vi "Bead threshold manual adjust 2.vi"(6 "Standalone(F)":bool, 7 "error in (no error)":errorcluster, 10 "Image In":T3) -> (0 "error out":errorcluster, 1 "enclosure box":T1 {"Rotation" format="%.2f"; "Left" scale=0.0..1024.0; "Right" scale=0.0..1024.0}, 2 "Centroid array":T4(array[cluster]), 3 "Source Image":T3(plugin-control) caption="Threshold Image")   [LabVIEW 2020]
uses:
  <vilib>/vision/Image Controls.llb/IMAQ Image.ctl
  <vilib>/vision/NI_Vision_Development_Module.lvlib
panel:
  out "Histogram":T2(graph)
  out "error out 2":errorcluster
  in  "Boundary":i16
  out "Centroid":cluster{"X Centroid":sgl, "Y Centroid":sgl} {"Y Centroid" format="%.2f"; "X Centroid" format="%.2f"}
  out "Reference Rectangles":i16[][](array[numeric])
  out "Number of Particles":i32
  in  "Morphology Iterations":i32=1
  in  "Morphology Operation":T5(ring)=enum."Erode"
  in  "Adjust Separation":i32=3 min=3
  in  "Threshold":cluster{sgl, sgl}(slide)={0.0, 168.81285} scale=0.0..255.0
  out "Color Palette out":cluster{"Red":u8, "Green":u8, "Blue":u8}[](array[cluster])
  in  "File Path":path
  in  "stop":bool
  out "Image Show Binary":T3(plugin-control)
  out "Selected Rectangle":i16[](array[numeric])
  out "Image Pixels (I16)":i16[][](array[numeric])
  out "Image Pixels (U8)":u8[][](array[numeric])
  out "Image Pixels (Float)":sgl[][](array[numeric]) format="%.2f"
  out "Image Pixels (U16)":u16[][](array[numeric])
  out "Source Image":T3(plugin-control) caption="Threshold Image"
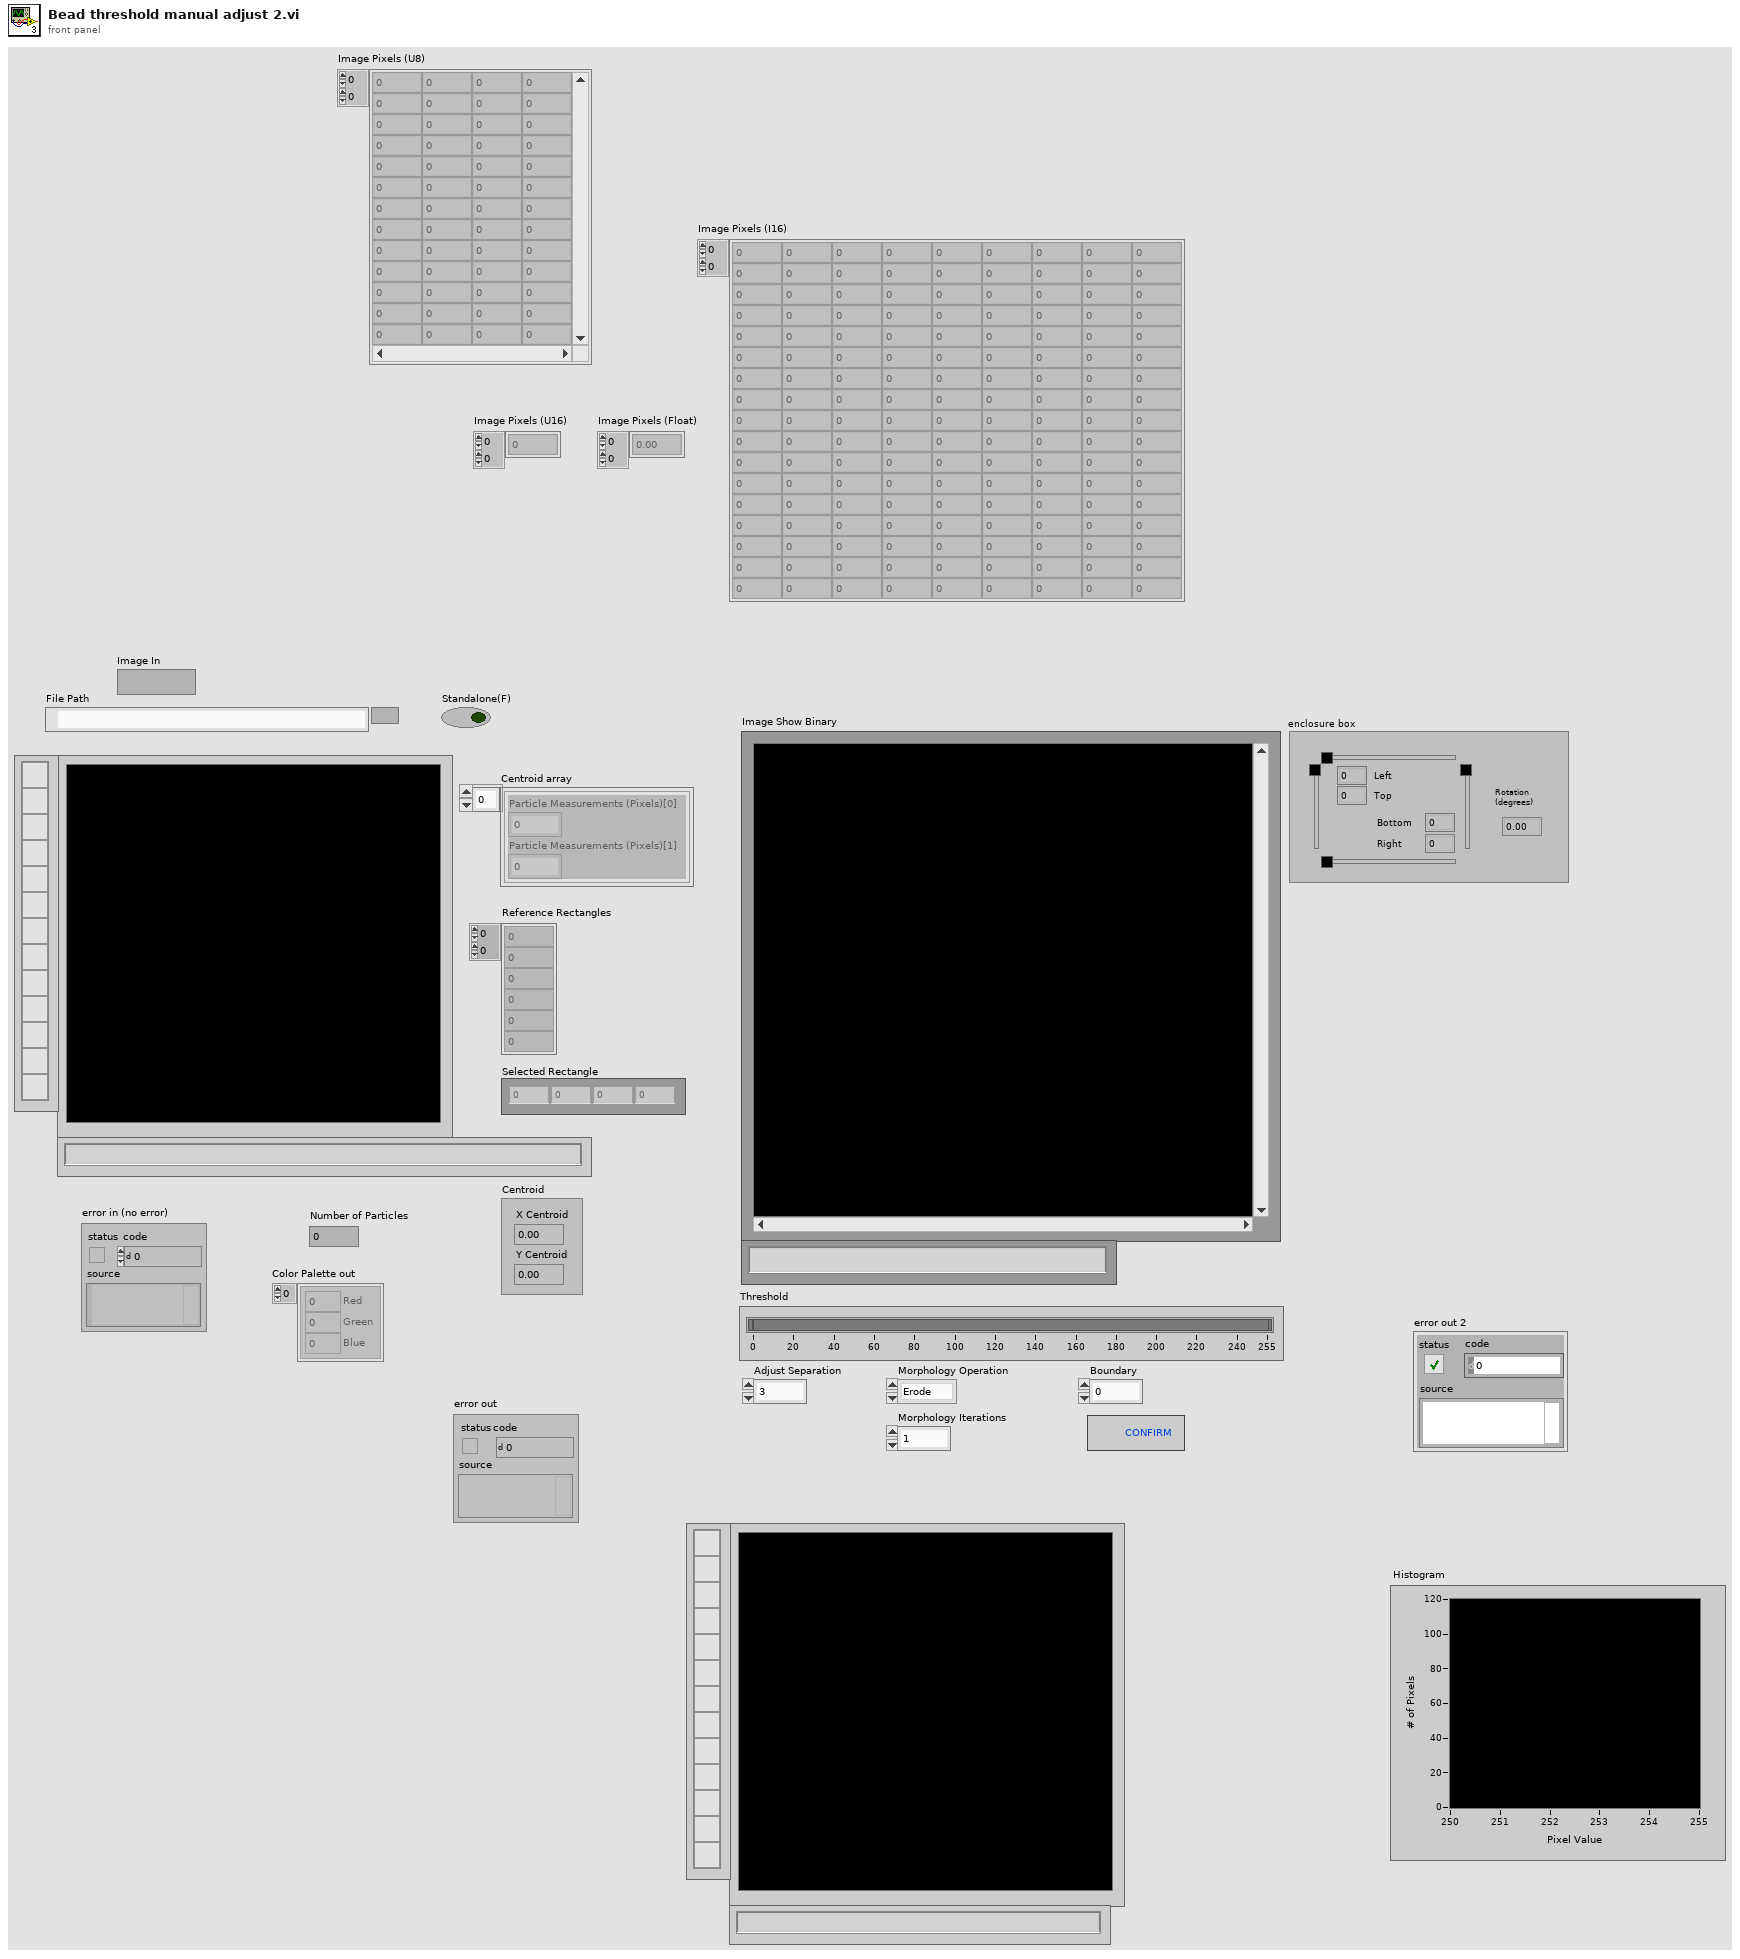
[diagram p1: front panel]
types:
  T1 = typedef "IMAQ Rectangle" = cluster{"Left":i32, "Top":i32, "Right":i32, "Bottom":i32, "Rotation":dbl}
  T2 = cluster{"Starting Value":sgl, "Incremental Value":sgl, "Histogram":u32[]}
  T3 = typedef "IMAQ Image.ctl" = refnum<image>
  T4 = cluster{"Particle Measurements (Pixels)[0]":dbl, "Particle Measurements (Pixels)[1]":dbl}[]
  T5 = enum32{"AutoM", "Close", "Dilate", "Erode", "Gradient", "Gradient out", "Gradient in", "Hit miss", "Open", "PClose", "POpen", "Thick", "Thin"}
  T6 = typedef "Image Type" = u32
  T7 = cluster{"Global Rectangle":i32[], "Contours":cluster{"Contour Type":u32, "ROI Type":u32, "Points":i32[]}[]}
  T8 = cluster{"Left":i32, "Top":i32, "Right":i32, "Bottom":i32}
  T9 = cluster{"Particle Measurements (Pixels)[0]":dbl, "Particle Measurements (Pixels)[1]":dbl}
  T10 = typedef "Particle Parameters" = i32
  T11 = typedef "ROI Descriptor" = cluster{"Global Rectangle":i32[], "Contours":cluster{"ID":enum32{"External", "Internal"}, "Type":u32, "Coordinates":i32[]}[]}
  T12 = cluster{"Measurement Parameter":T10, "Range Lower Value":dbl, "Range Upper Value":dbl, "Range":bool, "Measurement Type":bool}
  T13 = cluster{"Measurement Parameter":T10, "Range Lower Value":dbl, "Range Upper Value":dbl, "Range":bool, "Measurement Type":bool}[]
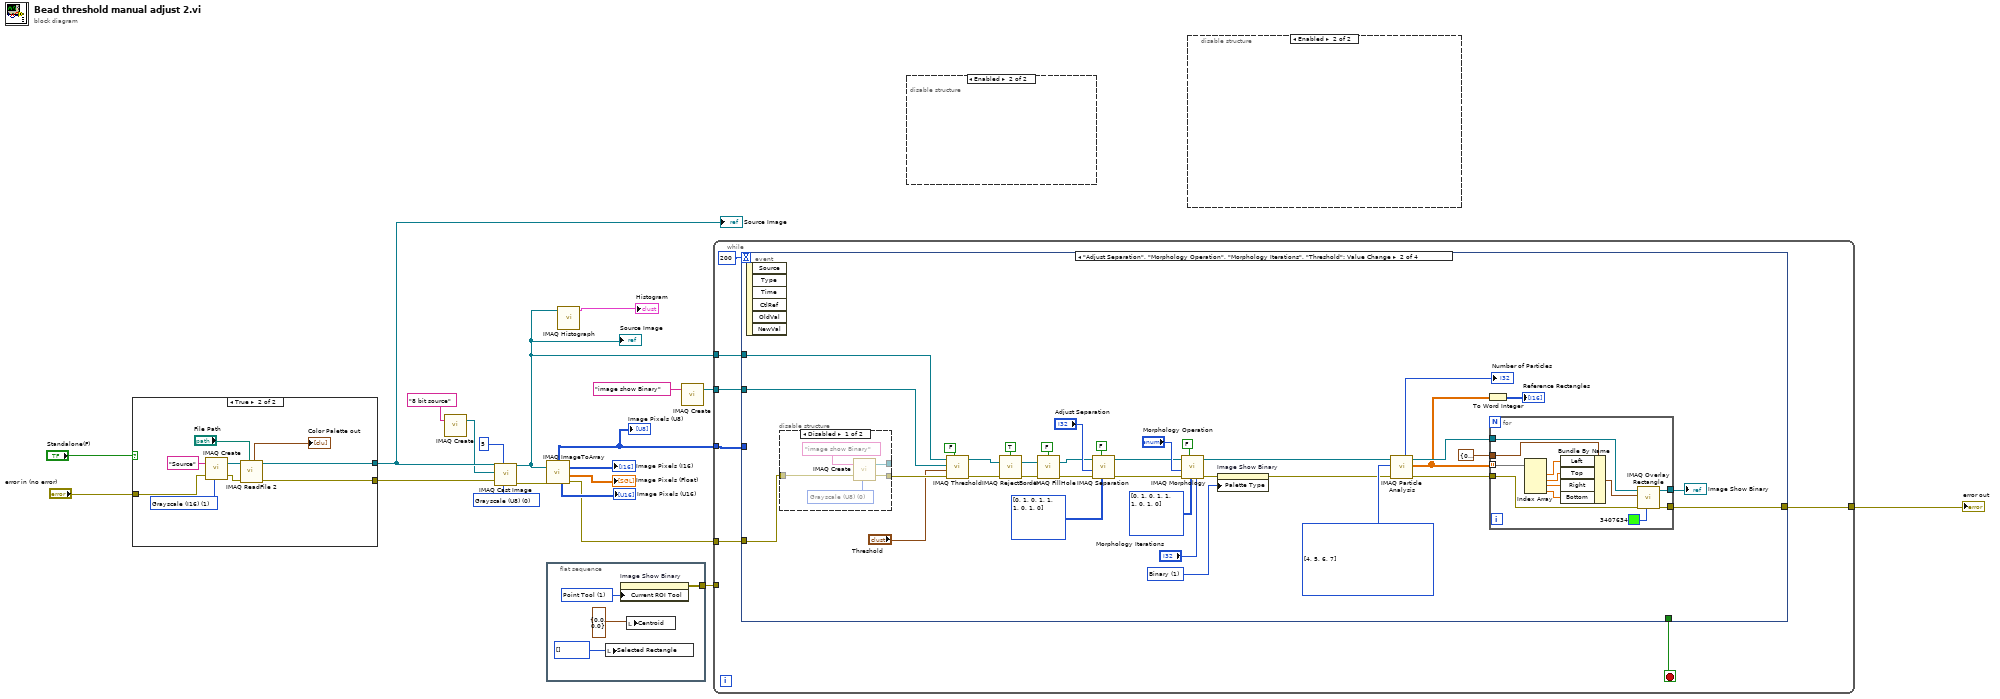
[diagram p0: block diagram]
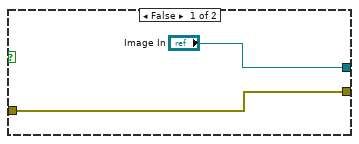
[diagram p2: hidden frame]
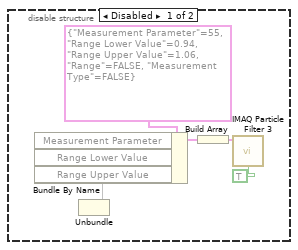
[diagram p3: hidden frame]
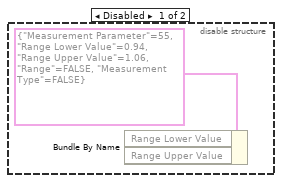
[diagram p4: hidden frame]
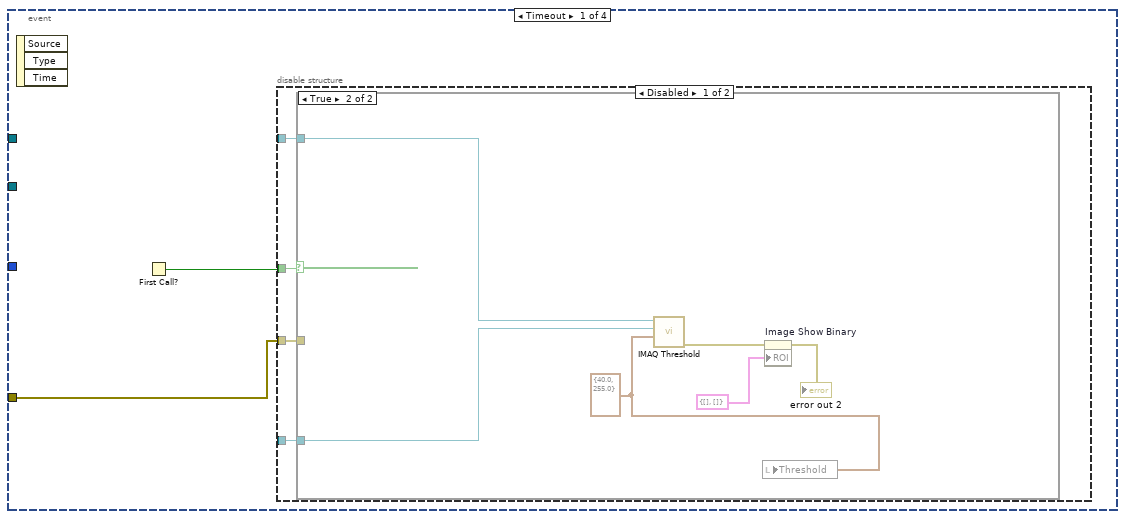
[diagram p5: hidden frame]
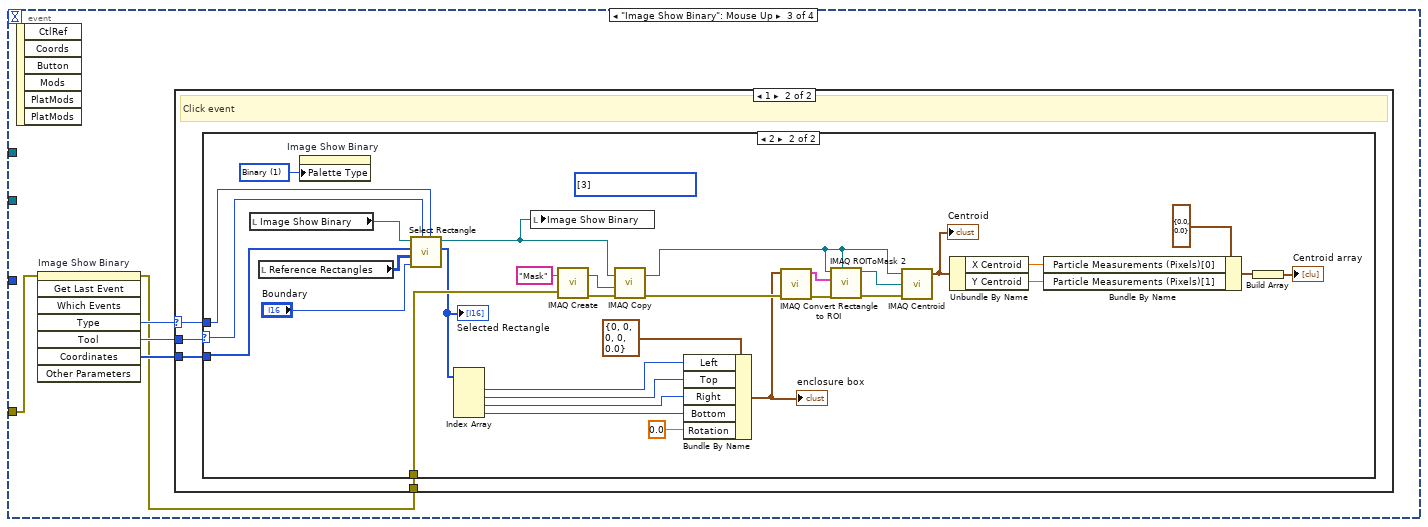
[diagram p9: hidden frame]
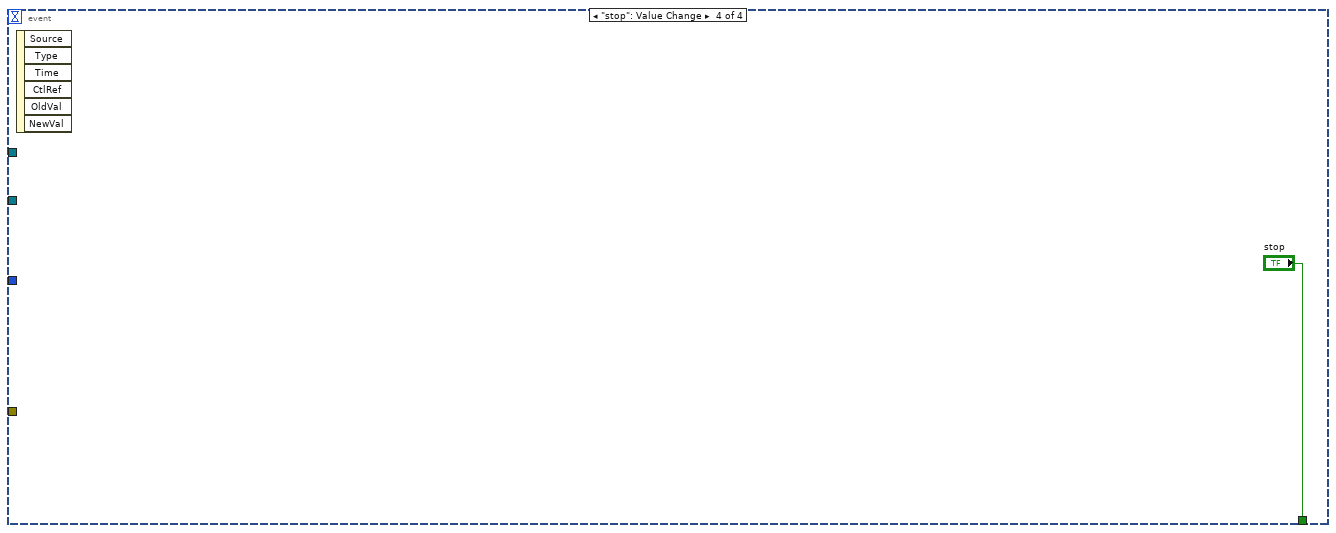
[diagram p12: hidden frame]
diagram:
  w7 = T6 0 items=["Grayscale (U8)", "Grayscale (I16)", "Grayscale (SGL)", "Complex (CSG)", "RGB (U32)", "HSL (U32)", "RGB (U64)", "Grayscale (U16)"] ("Image Type")
  n1 = case shown="True" "Standalone(F)" {
    tunnel: ["Image In" w24] -> w8
    tunnel: "error in (no error)" -> [w22 w25]
    tunnel: [w22 w23] -> w10
    frame False {
    }
    frame True {
      w31 = T6 1 items=["Grayscale (U8)", "Grayscale (I16)", "Grayscale (SGL)", "Complex (CSG)", "RGB (U32)", "HSL (U32)", "RGB (U64)", "Grayscale (U16)"] ("Image Type")
      n2 = call "IMAQ Create"("Image Name"="Source", "Image Type"=w31, "error in (no error)"=w25) -> ("New Image"=w29:T3, "error out"=w26:errorcluster)  [unwired: 2 in]
      n3 = call "IMAQ ReadFile 2"("File Path"="File Path", "error in (no error)"=w26, "Image"=w29) -> ("error out"=w23:errorcluster, "Image Out"=w24:T3, "Color Palette out"=→"Color Palette out":cluster{"Red":u8, "Green":u8, "Blue":u8}[])  [unwired: 4 in, 2 out]
    }
  }
  "Source Image" <- w8
  n4 = call "IMAQ Create"("Image Name"="8 bit source") -> ("New Image"=w2:T3)  [unwired: 4 in, 1 out]
  n5 = call "IMAQ Cast Image"("Image Type"=w7, "# Shifts"=5, "error in (no error)"=w10, "Image Dst"=w2, "Image Src"=w8) -> ("error out"=w9:errorcluster, "Image Dst Out"=w1:T3)  [unwired: 5 in]
  "Source Image" <- w1
  n6 = flat-sequence {
    tunnel: [w34] -> w12
    frame #0 {
      w35 = u32 1 items=["Zoom Tool"=8, "Selection Tool"=0, "Pan Tool"=9, "Point Tool"=1, "Line Tool"=2, "Rectangle Tool"=3, "Rotated Rectangle Tool"=12, "Polyline Tool"=10, "Polygon Tool"=5, "Freehand Tool"=11, "Closed Freehand Tool"=6, "Ellipse Tool"=4, "Annulus Tool"=7] ("Current ROI Tool")
      n7 = local write "Selected Rectangle"(i16[] []) -> ()
      n8 = property on="Image Show Binary" class="ImageControl"("Current ROI Tool"=w35) -> (error out=w34:errorcluster)  [unwired: 2 in, 1 out]
      n9 = local write "Centroid"(cluster{"X Centroid":sgl, "Y Centroid":sgl} {"X Centroid"=0.0, "Y Centroid"=0.0} ("Centroid")) -> ()
    }
  }
  n10 = call "IMAQ ImageToArray"("error in (no error)"=w9, "Image"=w1) -> ("Image Pixels (U16)"=→"Image Pixels (U16)":u16[][], "Image Pixels (Float)"=→"Image Pixels (Float)":sgl[][], "error out"=w15:errorcluster, "Image Pixels (U8)"=w17:u8[][], "Image Pixels (I16)"=→"Image Pixels (I16)":i16[][])  [unwired: 2 in]
  "Image Pixels (U8)" <- w17
  n11 = call "IMAQ Histograph"("Image"=w1) -> ("Histogram Graph"=→"Histogram":T2)  [unwired: 7 in, 3 out]
  n12 = call "IMAQ Create"("Image Name"="image show Binary") -> ("New Image"=w4:T3)  [unwired: 4 in, 1 out]
  n13 = while {
    tunnel: w17 -> [w42]
    tunnel: w1 -> [w39]
    tunnel: [w38] -> w16
    tunnel: w15 -> [w37]
    tunnel: w12 -> [_]
    tunnel: w4 -> [w36]
    stop <- w41 stop-if-true
    n14 = event shown="[1] \"Adjust Separation\", \"Morphology Operation\", \"Morphology Iterations\", \"Threshold\": Value Change" {
      selector: _ -> [_ _ _ _]
      dyn-events: _ -> [_ _ _ _]
      timeout: 200 -> [_ _ _ _]
      tunnel: w42 -> [_ _ _ _]
      tunnel: [_ _ _ "stop"] -> w41
      tunnel: w39 -> [_ w58 _ _]
      tunnel: [_ w63 _ _] -> w38
      tunnel: w37 -> [w43 w62 w110 _]
      tunnel: w36 -> [_ w57 _ _]
      event Timeout {
        n15 = event-data() -> ()  [unwired: 1 in, 3 out]
        n16 = First Call?() -> (First Call?: T/F=w44:bool)
        n17 = disable-structure shown="Disabled" {
          disable-tunnel: w44 -> [w48 _]
          disable-tunnel: _ -> [w47 _]
          disable-tunnel: w43 -> [w46 _]
          disable-tunnel: _ -> [w45 _]
          frame Disabled {
            n18 = case shown="True" w48 {
              tunnel: w47 -> [_ w50]
              tunnel: w46 -> [_ _]
              tunnel: w45 -> [_ w49]
              frame False {
              }
              frame True {
                w51 = cluster{"Lower value":sgl, "Upper value":sgl} {"Lower value"=40.0, "Upper value"=255.0} ("Range")
                n19 = call "IMAQ Threshold"("Range"=w51, "Image Dst"=w49, "Image Src"=w50) -> ("error out"=w53:errorcluster)  [unwired: 7 in, 1 out]
                n20 = local write "Threshold"(w51) -> ()
                n21 = property on="Image Show Binary" class="ImageControl"(error in=w53, "ROI"=T7 {"Global Rectangle"=[], "Contours"=[]}) -> (error out=→"error out 2":errorcluster)  [unwired: 1 in, 1 out]
              }
            }
          }
          frame Enabled {
          }
        }
      }
      event "Adjust Separation", "Morphology Operation", "Morphology Iterations", "Threshold": Value Change {
        w76 = T10[] [4, 5, 6, 7] items=["Center of Mass X", "Center of Mass Y", "First Pixel X", "First Pixel Y", "Bounding Rect Left", "Bounding Rect Top", "Bounding Rect Right", "Bounding Rect Bottom", "Max Feret Diameter Start X", "Max Feret Diameter Start Y", "Max Feret Diameter End X", "Max Feret Diameter End Y", "Max Horiz. Segment Length Left", "Max Horiz. Segment Length Right", "Max Horiz. Segment Length Row", "-", "Bounding Rect Width", "Bounding Rect Height", "Bounding Rect Diagonal", "Perimeter", "Convex Hull Perimeter", "Holes' Perimeter", "Max Feret Diameter", "Equivalent Ellipse Major Axis", "Equivalent Ellipse Minor Axis", "Equivalent Ellipse Minor Axis (Feret)", "Equivalent Rect Long Side", "Equivalent Rect Short Side", "Equivalent Rect Diagonal", "Equivalent Rect Short Side (Feret)", "Average Horiz. Segment Length", "Average Vert. Segment Length", "Hydraulic Radius", "Waddel Disk Diameter", "-", "Area", "Holes' Area", "Particle & Holes' Area", "Convex Hull Area", "Image Area", "-", "Number of Holes", "Number of Horiz. Segments", "Number of Vert. Segments", "-", "Orientation", "Max Feret Diameter Orientation", "-", "% Area/Image Area", "% Area/(Particle & Holes' Area)", "Ratio of Equivalent Ellipse Axes", "Ratio of Equivalent Rect Sides", "-", "Elongation Factor", "Compactness Factor", "Heywood Circularity Factor", "Type Factor", "-", "Sum X", "Sum Y", "Sum XX", "Sum XY", "Sum YY", "Sum XXX", "Sum XXY", "Sum XYY", "Sum YYY", "-", "Moment of Inertia XX", "Moment of Inertia XY", "Moment of Inertia YY", "Moment of Inertia XXX", "Moment of Inertia XXY", "Moment of Inertia XYY", "Moment of Inertia YYY", "Norm. Moment of Inertia XX", "Norm. Moment of Inertia XY", "Norm. Moment of Inertia YY", "Norm. Moment of Inertia XXX", "Norm. Moment of Inertia XXY", "Norm. Moment of Inertia XYY", "Norm. Moment of Inertia YYY", "Hu Moment 1", "Hu Moment 2", "Hu Moment 3", "Hu Moment 4", "Hu Moment 5", "Hu Moment 6", "Hu Moment 7"] ("Pixel Measurements")
        w78 = u32 1 items=["Grayscale", "Binary", "Gradient", "Rainbow", "Temperature", "User Defined", "Binary 16 Bit", "Gradient 16 Bit", "Rainbow 16 Bit", "Temperature 16 Bit", "User Defined 16 Bit"] ("Palette Type")
        n22 = event-data() -> ()  [unwired: 1 in, 6 out]
        n23 = disable-structure shown="Disabled" {
          disable-tunnel: w62 -> [w93 w96]
          disable-tunnel: [w92 _] -> _
          disable-tunnel: [w91 w96] -> w56
          frame Disabled {
            w94 = T6 0 items=["Grayscale (U8)", "Grayscale (I16)", "Grayscale (SGL)", "Complex (CSG)", "RGB (U32)", "HSL (U32)", "RGB (U64)", "Grayscale (U16)"] ("Image Type")
            n24 = call "IMAQ Create"("Image Name"="image show Binary", "Image Type"=w94, "error in (no error)"=w93) -> ("New Image"=w92:T3, "error out"=w91:errorcluster)  [unwired: 2 in]
          }
          frame Enabled {
          }
        }
        n25 = call "IMAQ Threshold"("Keep/Replace Value (Replace)"=FALSE, "error in (no error)"=w56, "Range"="Threshold", "Image Dst"=w57, "Image Src"=w58) -> ("error out"=w79:errorcluster, "Image Dst Out"=w67:T3)  [unwired: 5 in]
        n26 = call "IMAQ RejectBorder"("error in (no error)"=w79, "Image Src"=w67, "Connectivity 4/8 (8)"=TRUE) -> ("error out"=w89:errorcluster, "Image Dst Out"=w66:T3)  [unwired: 1 in, 2 out]
        n27 = call "IMAQ FillHole"("error in (no error)"=w89, "Image Src"=w66, "Connectivity 4/8 (8)"=FALSE) -> ("error out"=w85:errorcluster, "Image Dst Out"=w65:T3)  [unwired: 1 in, 2 out]
        n28 = call "IMAQ Separation"("Structuring Element"=i32[][] [[0, 1, 0], [1, 1, 1], [0, 1, 0]], "Square/Hexa (Square)"=FALSE, "error in (no error)"=w85, "Nb of Erosion"="Adjust Separation", "Image Src"=w65) -> ("error out"=w80:errorcluster, "Image Dst Out"=w64:T3)  [unwired: 1 in, 4 out]
        n29 = call "IMAQ Morphology"("Number of iterations (1)"="Morphology Iterations", "Structuring Element"=i32[][] [[0, 1, 0], [1, 1, 1], [0, 1, 0]], "Square/Hexa (Square)"=FALSE, "error in (no error)"=w80, "Operation"="Morphology Operation", "Image Src"=w64) -> ("error out"=w77:errorcluster, "Image Dst Out"=w68:T3)  [unwired: 1 in, 3 out]
        n30 = property on="Image Show Binary" class="ImageControl"(error in=w77, "Palette Type"=w78) -> (error out=w69:errorcluster)  [unwired: 1 in, 1 out]
        n31 = call "IMAQ Particle Analysis"("error in (no error)"=w69, "Pixel Measurements"=w76, "Image"=w68) -> ("error out"=w72:errorcluster, "Particle Measurements (Pixels)"=w71:dbl[][], "Image Out (duplicate)"=w75:T3, "Number of Particles"=→"Number of Particles":i32)  [unwired: 3 in, 2 out]
        n32 = To Word Integer(number=w71) -> (16bit integer=→"Reference Rectangles":i16[][])
        n33 = for {
          tunnel: [w99] -> w61
          tunnel: w75 -> [w107]
          tunnel: w71 -> [w105] mode=indexing
          tunnel: T8 {"Left"=0, "Top"=0, "Right"=0, "Bottom"=0} ("Rectangle") -> [w106]
          tunnel: [w98] -> w63
          tunnel: w72 -> [w97]
          n34 = Index Array(array=w105) -> (element #1=w103:dbl, element #2=w102:dbl, element #3=w101:dbl, element #4=w100:dbl)  [unwired: 4 in]
          n35 = Bundle By Name(cluster=w106, "Left"=w103, "Top"=w102, "Right"=w101, "Bottom"=w100) -> (w104:T8)
          n36 = call "IMAQ Overlay Rectangle"("Color"=u32 3407634 ("Text Color (black)"), "error in (no error)"=w97, "Rectangle"=w104, "Image"=w107) -> ("error out"=w98:errorcluster, "Image Out"=w99:T3)  [unwired: 6 in]
        }
        "Image Show Binary" <- w61
      }
      event "Image Show Binary": Mouse Up {
        n37 = event-data() -> ()  [unwired: 1 in, 6 out]
        n38 = invoke on="Image Show Binary" class="ImageControl" method="Get Last Event"(error in=w110) -> (error out=w109:errorcluster, "Type"=w113:i32, "Tool"=w112:i32, "Coordinates"=w111:i32[])  [unwired: 7 in, 4 out]
        n39 = case shown="1" w113 {
          selector: w113 -> [_ w116]
          tunnel: w112 -> [_ w117]
          tunnel: w111 -> [_ w115]
          tunnel: w109 -> [_ w114]
          frame 0, Default {
          }
          frame 1 {
            # "Click event"
            n40 = case shown="2" w117 {
              selector: w117 -> [_ w147]
              tunnel: w116 -> [_ w148]
              tunnel: w115 -> [_ w146]
              tunnel: w114 -> [_ w133]
              frame 0, Default {
              }
              frame 2 {
                (unwired) u32[] [3] items=["No Selection", "Point", "Line", "Rectangle", "Oval", "Polygon", "Freehand Region", "Annulus", "Zoom", "Pan", "Broken Line", "Freehand Line", "Rotated Rectangle"] ("Tools")
                w145 = u32 1 items=["Grayscale", "Binary", "Gradient", "Rainbow", "Temperature", "User Defined", "Binary 16 Bit", "Gradient 16 Bit", "Rainbow 16 Bit", "Temperature 16 Bit", "User Defined 16 Bit"] ("Palette:Palette Type")
                n41 = local read "Image Show Binary"() -> (w149:T3)
                n42 = local read "Reference Rectangles"() -> (w144:i16[][])
                n43 = property on="Image Show Binary" class="ImageControl"("Palette Type"=w145) -> ()  [unwired: 2 in, 2 out]
                n44 = call "Select Rectangle.vi"("Type"=w148, "Tool"=w147, "Boundary"="Boundary", "Reference Rectangle"=w144, "Coordinates"=w146, "Image In"=w149) -> ("Selected Reference Rectangle"=w129:i16[], "Image Out"=w140:T3)  [unwired: 2 in, 2 out]
                "Selected Rectangle" <- w129
                n45 = Index Array(array=w129) -> (element #1=w128:i16, element #2=w127:i16, element #3=w126:i16, element #4=w125:i16)  [unwired: 4 in]
                n46 = local write "Image Show Binary"(w140) -> ()
                n47 = call "IMAQ Create"("Image Name"="Mask", "error in (no error)"=w133) -> ("New Image"=w141:T3, "error out"=w142:errorcluster)  [unwired: 3 in]
                n48 = call "IMAQ Copy"("error in (no error)"=w142, "Image Dst"=w141, "Image Src"=w140) -> ("error out"=w132:errorcluster, "Image Dst Out"=w120:T3)  [unwired: 3 in]
                n49 = Bundle By Name(cluster=T1 {"Left"=0, "Top"=0, "Right"=0, "Bottom"=0, "Rotation"=0.0} ("Rectangle"), "Left"=w128, "Top"=w127, "Right"=w126, "Bottom"=w125, "Rotation"=0.0) -> (w124:T1)
                "enclosure box" <- w124
                n50 = call "IMAQ Convert Rectangle to ROI"("error in (no error)"=w132, "Rectangle"=w124) -> ("error out"=w123:errorcluster, "ROI Descriptor"=w122:T11)  [unwired: 7 in]
                n51 = call "IMAQ ROIToMask 2"("Image Model"=w120, "error in (no error)"=w123, "ROI Descriptor"=w122, "Image"=w120) -> ("error out"=w138:errorcluster, "Image Out"=w121:T3)  [unwired: 5 in, 1 out]
                n52 = call "IMAQ Centroid"("error in (no error)"=w138, "Image Mask"=w121, "Image"=w120) -> ("Centroid"=w139:cluster{"X Centroid":sgl, "Y Centroid":sgl})  [unwired: 1 in, 1 out]
                "Centroid" <- w139
                n53 = Unbundle By Name(w139) -> ("X Centroid"=w136:sgl, "Y Centroid"=w135:sgl)
                n54 = Bundle By Name(cluster=T9 {"Particle Measurements (Pixels)[0]"=0.0, "Particle Measurements (Pixels)[1]"=0.0}, "Particle Measurements (Pixels)[0]"=w136, "Particle Measurements (Pixels)[1]"=w135) -> (w119:T9)
                n55 = Build Array(w119) -> (→"Centroid array":T4)
              }
            }
          }
        }
      }
      event "stop": Value Change {
        n56 = event-data() -> ()  [unwired: 1 in, 6 out]
      }
    }
  }
  "error out" <- w16
  n57 = disable-structure shown="Enabled" {
    frame Disabled {
      n58 = Bundle By Name(cluster=T12 {"Measurement Parameter"=55, "Range Lower Value"=0.94, "Range Upper Value"=1.06, "Range"=FALSE, "Measurement Type"=FALSE} ("Selection Value")) -> ()  [unwired: 2 in, 1 out]
    }
    frame Enabled {
    }
  }
  n59 = disable-structure shown="Enabled" {
    frame Disabled {
      n60 = Unbundle() -> (w154:cluster{sgl, sgl}, w155, w156)
      n61 = Bundle By Name(cluster=T12 {"Measurement Parameter"=55, "Range Lower Value"=0.94, "Range Upper Value"=1.06, "Range"=FALSE, "Measurement Type"=FALSE} ("Selection Value"), "Range Lower Value"=w155, "Range Upper Value"=w156) -> (w157:T12, "Measurement Parameter"=w159:T10)
      n62 = Build Array(w157) -> (w158:T13)
      n63 = call "IMAQ Particle Filter 3"("Selection Values"=w158, "Fill Holes? (F)"=TRUE) -> ()  [unwired: 11 in, 3 out]
    }
    frame Enabled {
    }
  }
